vi "Get Connected.vi"(8 "error in (no error)":errorcluster, 11 "TCP Client in":refnum<class "TCP Client.lvclass">) -> (0 "error out":errorcluster, 2 "Connected":bool, 3 "TCP Client out":refnum<class "TCP Client.lvclass">)   [LabVIEW 2020, in "Stream-TCP.lvlib" / "TCP Client.lvclass"]
uses:
  TCP Client.lvclass
  Connection State.ctl
  TCP Client.lvclass/TCP Client.ctl
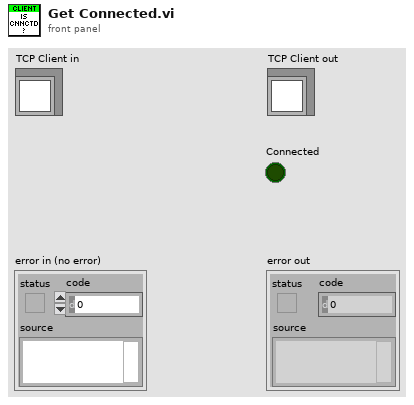
[diagram p1: front panel]
types:
  T1 = typedef "Stream-TCP.lvlib/TCP Client.lvclass/Connection State.ctl" = enum16{"Closed", "Idle", "Connecting", "Connected", "Shutdown"}
  T2 = typedef "Stream-TCP.lvlib/TCP Client.lvclass/Ref Data.ctl" = cluster{"TCP Connection":refnum<k5>, "TCP Stream":refnum<class "TCP Stream.lvclass">, "State":T1, "Connection Loop":refnum<vi>, "TCP Mode":T3, "Timeout ms":i32, "Server Connection":bool}
  T3 = typedef "Stream-TCP.lvlib/TCP Mode.ctl" = enum16{"buffered", "raw"}
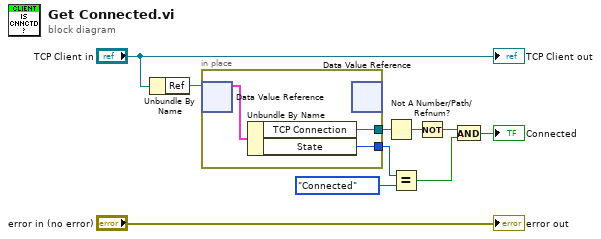
[diagram p0: block diagram]
diagram:
  n1 = Unbundle By Name("TCP Client in") -> ("Ref"=w10:refnum<data-value>)
  n2 = in-place {
    in-place-border: [w12] -> w9
    in-place-border: [w11] -> w7
    n3 = in-place-dvr #1(w10) -> (w13:T2)  [unwired: 1 out]
    n4 = Unbundle By Name(w13) -> ("TCP Connection"=w12:refnum<k5>, "State"=w11:T1)
    n5 = in-place-dvr #1() -> ()  [unwired: 1 in, 2 out]
  }
  n6 = Not A Number/Path/Refnum?(number/path/refnum=w9) -> (NaN/Path/Refnum?=w8:bool)
  n7 = Equal?(x=w7, y=Connection_State."Connected") -> (x = y?=w4:bool)
  n8 = Not(x=w8) -> (.not. x?=w5:bool)
  n9 = And(x=w5, y=w4) -> (x .and. y?=→"Connected":bool)
  "error out" <- "error in (no error)"
  "TCP Client out" <- "TCP Client in"
